vi "DAQmx多通道单点输出.vi"() -> ()   [LabVIEW 2010]
uses:
  <vilib>/DAQmx/write.llb/DAQmx Write.vi
  <vilib>/DAQmx/write.llb/DAQmx Write (Analog 1D DBL NChan 1Samp).vi
  <vilib>/DAQmx/create/channels.llb/DAQmx Create Channel (AO-Voltage-Basic).vi
  <vilib>/daqmx/miscellaneous.llb/DAQmx Fill In Error Info.vi
panel:
  out "error out":errorcluster
  in  "data":dbl[](array[numeric])=[1.0, -1.0] format="%0.2f"
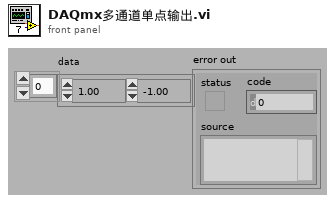
[diagram p1: front panel]
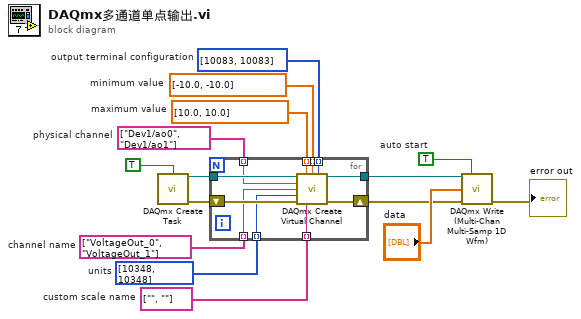
[diagram p0: block diagram]
diagram:
  w5 = i32[] [10083, 10083] items=["Default"=-1, "RSE"=10083, "Differential"=10106, "Pseudodifferential"=12529]  # output terminal configuration
  w6 = string[] ["", ""]  # custom scale name
  w7 = i32[] [10348, 10348] items=["Volts"=10348, "From Custom Scale"=10065]  # units
  w8 = string[] ["VoltageOut_0", "VoltageOut_1"]  # channel name
  w9 = string[] ["Dev1/ao0", "Dev1/ao1"]  # physical channel
  w10 = dbl[] [10.0, 10.0]  # maximum value
  w11 = dbl[] [-10.0, -10.0]  # minimum value
  w15 = TRUE  # auto start
  n1 = call <vilib>:"DAQmx Create Task.vi"("auto cleanup"=TRUE) -> ("task out"=w13:refnum<k21>, "error out"=w12:errorcluster)  [unwired: 13 in]
  n2 = for "For循环" {
    tunnel: w13 -> [w26]
    tunnel: [w24] -> w3
    tunnel: w11 -> [w22] mode=indexing
    tunnel: w10 -> [w21] mode=indexing
    tunnel: w9 -> [w20] mode=indexing
    tunnel: w8 -> [w19] mode=indexing
    tunnel: w7 -> [w18] mode=indexing
    tunnel: w6 -> [w17] mode=indexing
    shift-right: [w23] -> w2
    shift-left: w12 -> [w25]
    tunnel: w5 -> [w16] mode=indexing
    n3 = call-poly <vilib>:"DAQmx Create Virtual Channel.vi"("task in"=w26, "maximum value"=w21, "minimum value"=w22, "output terminal configuration"=w16, "physical channels"=w20, "name to assign"=w19, "units"=w18, "error in"=w25, "custom scale name"=w17) -> ("task out"=w24:refnum<k21>, "error out"=w23:errorcluster)  [unwired: 5 in]
  }
  n4 = call-poly "DAQmx Write (Multi-Chan Multi-Samp 1D Wfm).vi"("task/channels in"=w3, "auto start"=w15, "data"="data", "error in"=w2) -> ("error out"=→"error out":errorcluster)  [unwired: 9 in, 2 out]
